vi "Tag Larvae (SubVI).vi"(11 "Array in":i32[][](array[numeric])) -> (1 "Bounding Box":i32[][](array[numeric]), 2 "Current ID":i32[](array[numeric]), 3 "Current Table":i16[][](array[numeric]))   [LabVIEW 2020]
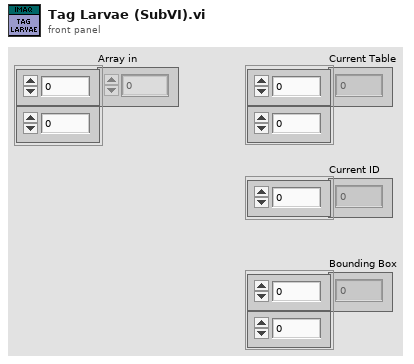
[diagram p1: front panel]
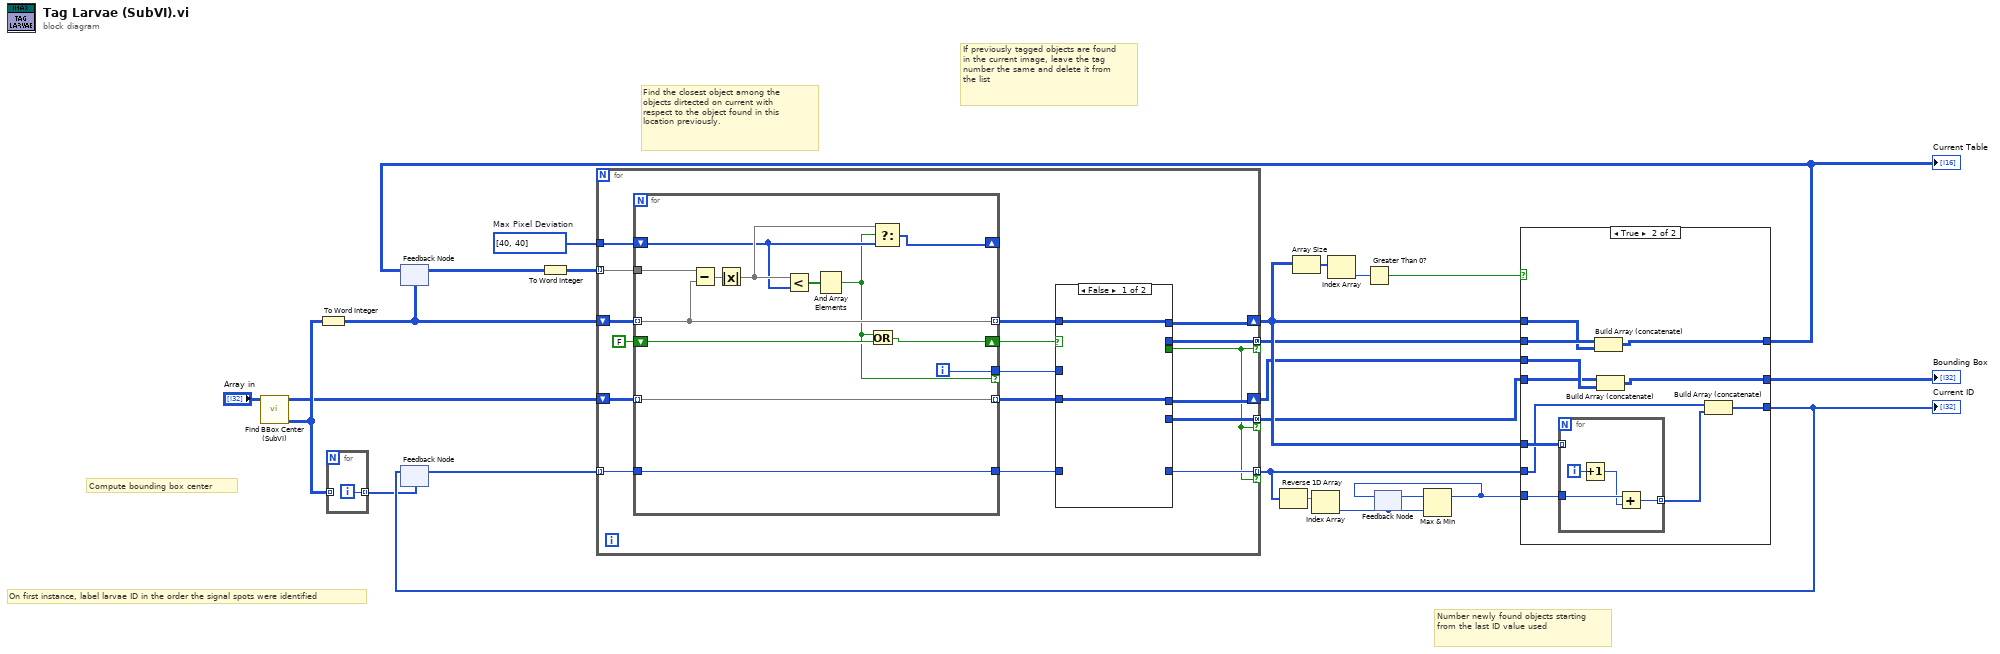
[diagram p0: block diagram]
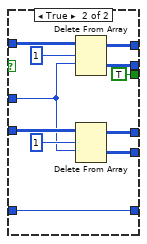
[diagram p3: hidden frame]
diagram:
  w9 = i16[] [40, 40]  # Max Pixel Deviation
  # "If previously tagged objects are found in the current image, leave the tag number the same and delete it from the list"
  # "Number newly found objects starting from the last ID value used"
  # "Find the closest object among the objects dirtected on current with respect to the object found in this location previously."
  # "On first instance, label larvae ID in the order the signal spots were identified"
  # "Compute bounding box center"
  n1 = call "Find BBox Center (SubVI).vi"("BBox Array In"="Array in") -> ("Center Array"=w3:i32[][], "BBox Array Out"=w2:i32[][])  [unwired: 9 in]
  n2 = To Word Integer(number=w3) -> (16bit integer=w11:i16[][])
  n3 = for {
    tunnel: w3 -> [_] mode=indexing
    tunnel: [w25] -> w12 mode=indexing
    i -> [w25]
  }
  n4 = feedback #1(w11) -> (w6:i16[][])
  n5 = feedback #2(w12) -> (w10:i32[])
  n6 = To Word Integer(number=w6) -> (16bit integer=w8:i16[][])
  n7 = for {
    tunnel: w8 -> [w42] mode=indexing
    shift-right: [w34] -> w17
    shift-left: w11 -> [w41]
    shift-right: [w33] -> w5
    shift-left: w2 -> [w40]
    tunnel: [w31] -> w16 mode=concatenating if=w26
    tunnel: [w30] -> w20 mode=indexing if=w26
    tunnel: w9 -> [w39]
    tunnel: [w27] -> w4 mode=concatenating if=w26
    tunnel: w10 -> [w36] mode=indexing
    n8 = for {
      tunnel: w42 -> [w68]
      tunnel: w41 -> [w63] mode=indexing
      tunnel: w40 -> [w60] mode=indexing
      shift-right: [w56] -> _
      shift-left: w39 -> [w65]
      tunnel: [w63] -> w38 mode=indexing
      shift-right: [w62] -> w29
      shift-left: FALSE -> [w61]
      tunnel: w36 -> [w57]
      tunnel: [w60] -> w35 mode=indexing
      tunnel: [w59] -> w32 if=w58
      tunnel: [w57] -> w28
      i -> [w59]
      n9 = Subtract(x=w68, y=w63) -> (x-y=w67:i16[])
      n10 = Absolute Value(x=w67) -> (abs(x)=w66:i16[])
      n11 = Less?(x=w66, y=w65) -> (x < y?=w64:bool[])
      n12 = And Array Elements(Boolean array=w64) -> (logical AND=w58:bool)
      n13 = Or(x=w58, y=w61) -> (x .or. y?=w62:bool)
      n14 = Select(t=w66, s=w58, f=w65) -> (s? t:f=w56:i16[])
    }
    n15 = case shown="False" w29 {
      tunnel: w38 -> [w44 w55]
      tunnel: w35 -> [w43 w54]
      tunnel: [w44 w53] -> w34
      tunnel: [w43 w52] -> w33
      tunnel: w28 -> [_ w45]
      tunnel: w32 -> [_ w46]
      tunnel: [_ w49] -> w31
      tunnel: [_ w45] -> w30
      tunnel: [_ TRUE] -> w26
      tunnel: [_ w47] -> w27
      frame False {
      }
      frame True {
        n16 = Delete From Array(array=w55, length=1, index (row)=w46) -> (deleted portion=w49:i16[][], array with subset deleted=w53:i16[][])  [unwired: 1 in]
        n17 = Delete From Array(array=w54, length=1, index (row)=w46) -> (deleted portion=w47:i32[][], array with subset deleted=w52:i32[][])  [unwired: 1 in]
      }
    }
  }
  n18 = Reverse 1D Array(array=w20) -> (reversed array=w21:i32[])
  n19 = Array Size(array=w17) -> (size(s)=w14:i32[])
  n20 = Index Array(array=w21) -> (element=w23:i32)  [unwired: 1 in]
  n21 = Index Array(array=w14) -> (element=w15:i32)  [unwired: 1 in]
  n22 = Greater Than 0?(x=w15) -> (x > 0?=w13:bool)
  n23 = feedback #3(w23) -> (w22:i32)
  n24 = Max & Min(x=w22, y=w23) -> (max(x,y)=w24:i32)  [unwired: 1 out]
  n25 = feedback-in #3(w24) -> ()
  n26 = case shown="True" w13 {
    tunnel: w20 -> [w71 w79]
    tunnel: [w71 w80] -> w19
    tunnel: w17 -> [_ w82]
    tunnel: w16 -> [w70 w78]
    tunnel: w17 -> [_ w77]
    tunnel: [w70 w76] -> w18
    tunnel: w24 -> [_ w75]
    tunnel: w4 -> [w69 w72]
    tunnel: w5 -> [_ w73]
    tunnel: [w69 w74] -> w1
    frame False {
    }
    frame True {
      n27 = for {
        tunnel: w82 -> [_] mode=indexing
        tunnel: w75 -> [w85]
        tunnel: [w86] -> w81 mode=indexing
        i -> [w84]
        n28 = Increment(x=w84) -> (x+1=w83:i32)
        n29 = Add(x=w85, y=w83) -> (x+y=w86:i32)
      }
      n30 = Build Array (concatenate)(w78, w77) -> (w76:i16[][])
      n31 = Build Array (concatenate)(w72, w73) -> (w74:i32[][])
      n32 = Build Array (concatenate)(w79, w81) -> (w80:i32[])
    }
  }
  "Current ID" <- w19
  "Current Table" <- w18
  "Bounding Box" <- w1
  n33 = feedback-in #1(w18) -> ()
  n34 = feedback-in #2(w19) -> ()
